vi "CloseClipboard.vi"(4 "error in (no error)":errorcluster) -> (0 "error out":errorcluster)   [LabVIEW 2011]
uses:
  KERNEL32.DLL
  user32.dll
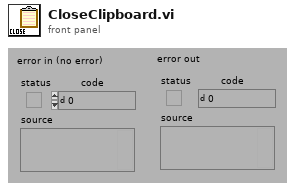
[diagram p1: front panel]
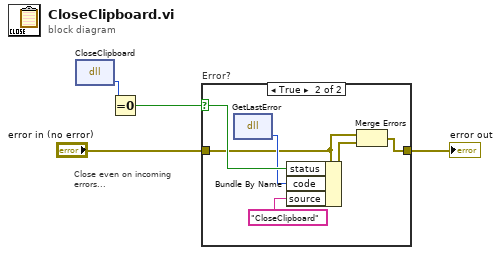
[diagram p0: block diagram]
diagram:
  # "Close even on incoming\nerrors..."
  n1 = dll-call lib="User32.dll" fn="CloseClipboard" label="unsigned long CloseClipboard(void);"() -> (w2:u32)  [unwired: 3 in, 2 out]
  n2 = Equal To 0?(x=w2) -> (x = 0?=w1:bool)
  n3 = case "Error?" shown="True" w1 {
    selector: w1 -> [_ w11]
    tunnel: "error in (no error)" -> [w5 w8]
    tunnel: [w5 w6] -> w4
    frame False {
    }
    frame True {
      n4 = dll-call lib="kernel32.dll" fn="GetLastError"() -> (w9:i32)  [unwired: 3 in, 2 out]
      n5 = Bundle By Name(cluster=w8, "status"=w11, "code"=w9, "source"="CloseClipboard") -> (w7:errorcluster)
      n6 = Merge Errors(w8, w7) -> (w6:errorcluster)
    }
  }
  "error out" <- w4
